vi "Merge Required Strings.vi"(0 "Strings In":string[](array[string]), 5 "Required":T1) -> (4 "Strings Out":string[](array[string]), 10 "Req'd":bool[](array[boolean]))   [LabVIEW 2020, in "KListboxEx.xctl"]
uses:
  KListboxEx.xctl
  Required.ctl
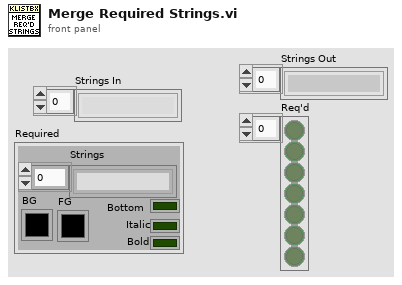
[diagram p1: front panel]
types:
  T1 = typedef "KListboxEx.xctl/Required.ctl" = cluster{"Strings":string[], "Bottom":bool, "Italic":bool, "FG":u32, "BG":u32, "Bold":bool}
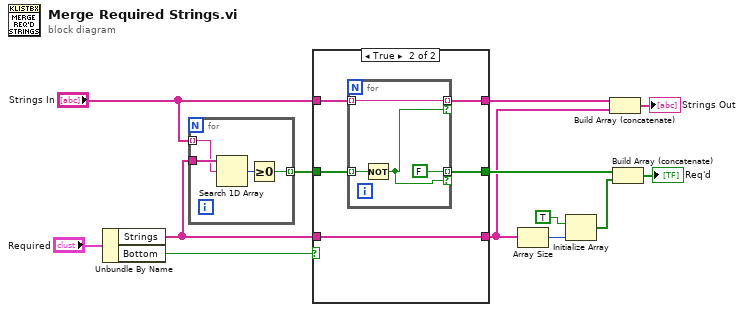
[diagram p0: block diagram]
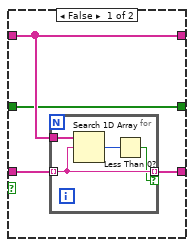
[diagram p2: hidden frame]
diagram:
  n1 = Unbundle By Name("Required") -> ("Strings"=w5:string[], "Bottom"=w3:bool)
  n2 = for {
    tunnel: w5 -> [w17]
    tunnel: "Strings In" -> [w15] mode=indexing
    tunnel: [w14] -> w6 mode=indexing
    n3 = Search 1D Array(1D array=w17, element=w15) -> (index of element=w16:i32)  [unwired: 1 in]
    n4 = Greater Or Equal To 0?(x=w16) -> (x >= 0?=w14:bool)
  }
  n5 = case shown="True" w3 {
    tunnel: w5 -> [w21 w26]
    tunnel: w6 -> [w19 w30]
    tunnel: "Strings In" -> [w20 w29]
    tunnel: [w20 w27] -> w11
    tunnel: [w19 w28] -> w13
    tunnel: [w18 w26] -> w12
    frame False {
      n6 = for {
        tunnel: w21 -> [w23] mode=indexing
        tunnel: w20 -> [w25]
        tunnel: [w23] -> w18 mode=indexing if=w22
        n7 = Search 1D Array(1D array=w25, element=w23) -> (index of element=w24:i32)  [unwired: 1 in]
        n8 = Less Than 0?(x=w24) -> (x < 0?=w22:bool)
      }
    }
    frame True {
      n9 = for {
        tunnel: w30 -> [w33] mode=indexing
        tunnel: w29 -> [w34] mode=indexing
        tunnel: [w34] -> w27 mode=indexing if=w31
        tunnel: [FALSE] -> w28 mode=indexing if=w31
        n10 = Not(x=w33) -> (.not. x?=w31:bool)
      }
    }
  }
  n11 = Array Size(array=w12) -> (size(s)=w10:i32)
  n12 = Initialize Array(TRUE, w10) -> (w8:bool[])
  n13 = Build Array (concatenate)(w11, w12) -> (→"Strings Out":string[])
  n14 = Build Array (concatenate)(w13, w8) -> (→"Req'd":bool[])
